vi "Enable Output.vi"(8 "error in (no error)":errorcluster, 9 "channel (1)":u8=1 min=1 max=4 step=1, 10 "output (T:on)":bool=TRUE, 11 "VISA resource name":refnum<visa-resource-name>) -> (0 "error out":errorcluster, 3 "VISA resource name out":refnum<visa-resource-name>)   [LabVIEW 2020, in "Agilent 6XXX Series.lvlib"]
doc: "This function enables or disables power supply output."
uses:
  <instrlib>/Agilent 6XXX Series/Agilent 6XXX Series.lvlib
panel:
  # "on\noff"
  # "*662xA only"
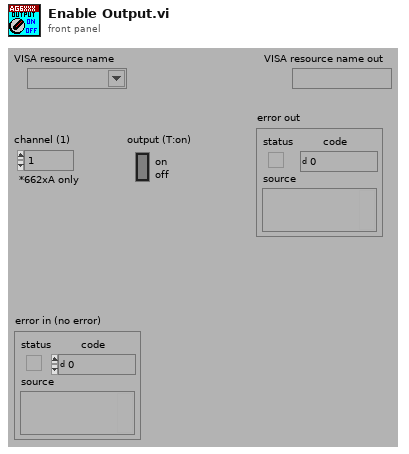
[diagram p1: front panel]
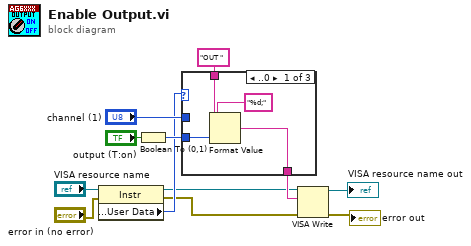
[diagram p0: block diagram]
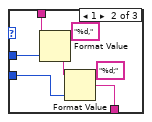
[diagram p2: hidden frame]
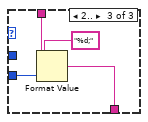
[diagram p3: hidden frame]
diagram:
  n1 = property class="Instr"(reference="VISA resource name", error in="error in (no error)") -> (reference out=w2:refnum<visa-resource-name>, error out=w1:errorcluster, "General Settings:User Data"=w3:u32)
  n2 = Boolean To (0,1)(Boolean="output (T:on)") -> (0, 1=w8:i16)
  n3 = case shown="..0" w3 {
    tunnel: "OUT " -> [w15 w22 w26]
    tunnel: w8 -> [w14 w18 w25]
    tunnel: "channel (1)" -> [_ w23 _]
    tunnel: [w13 w17 w24] -> w6
    frame ..0 {
      n4 = Format Value(string ("")=w15, format string="%d;", value (0)=w14) -> (output string=w13:string)
    }
    frame 1 {
      n5 = Format Value(string ("")=w22, format string="%d,", value (0)=w23) -> (output string=w19:string)
      n6 = Format Value(string ("")=w19, format string="%d;", value (0)=w18) -> (output string=w17:string)
    }
    frame 2.. {
      n7 = Format Value(string ("")=w26, format string="%d;", value (0)=w25) -> (output string=w24:string)
    }
  }
  n8 = VISA Write(VISA resource name=w2, write buffer=w6, error in (no error)=w1) -> (VISA resource name out=→"VISA resource name out":refnum<visa-resource-name>, error out=→"error out":errorcluster)  [unwired: 1 out]
